vi "azymut.vi"() -> ()   [LabVIEW 2015, in "Biblioteka moduł map v3.lvlib" / "Zmienne.lvlib"]
uses:
  Zmienne.lvlib
panel:
  in  "azymut":dbl
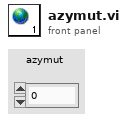
[diagram p1: front panel]
diagram:
